vi "ArrayToStr.vi"(1 "Array":string[](array[string])) -> (0 "Str":string)   [LabVIEW 2013]
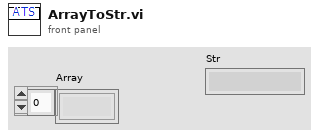
[diagram p1: front panel]
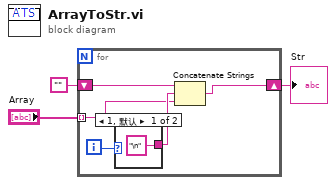
[diagram p0: block diagram]
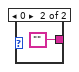
[diagram p2: hidden frame]
diagram:
  n1 = for {
    tunnel: "Array" -> [w5] mode=indexing
    shift-right: [w4] -> w1
    shift-left: "" -> [w8]
    i -> [w7]
    n2 = case shown="1, 默认" w7 {
      tunnel: ["\n" ""] -> w6
      frame 1, Default {
      }
      frame 0 {
      }
    }
    n3 = Concatenate Strings(w8, w6, w5) -> (w4:string)
  }
  "Str" <- w1
